vi "read config INI.vi"(8 "error in (no error)":errorcluster, 11 "Cluster in":refnum<vi>) -> (0 "error out":errorcluster, 3 "config.ini value":T1)   [LabVIEW 2014]
uses:
  <vilib>/Utility/config.llb/Read Key (Double).vi
  <vilib>/Utility/config.llb/NI_LVConfig.lvlib
panel:
  # "temperature"
  # "heater"
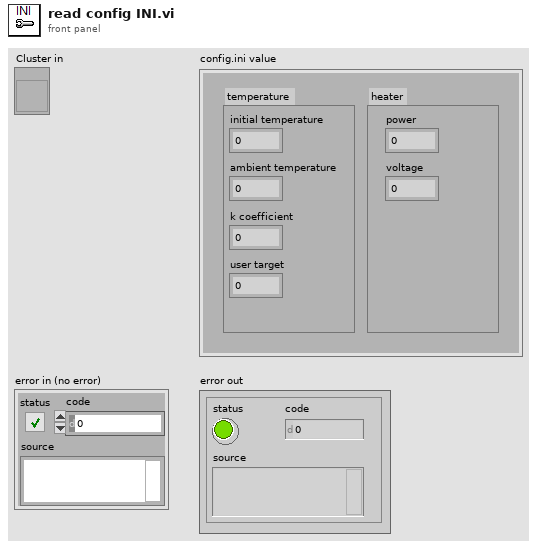
[diagram p1: front panel]
types:
  T1 = cluster{"initial temperature":sgl, "k coefficient":sgl, "ambient temperature":sgl, "user target ":sgl, "power":sgl, "voltage":sgl}
  T2 = typedef "NI_LVConfig.lvlib/Config Data RefNum.ctl" = refnum<k1>
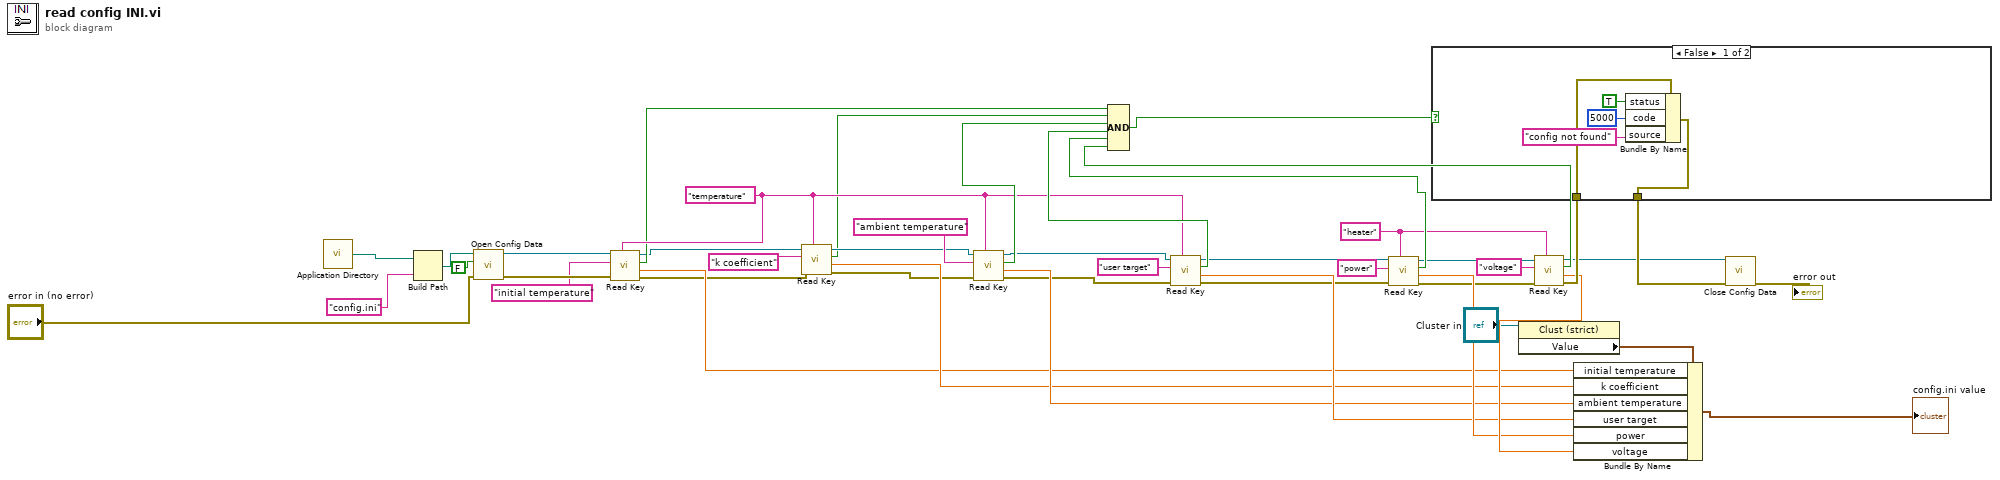
[diagram p0: block diagram]
diagram:
  w25 = "heater" ("section")
  w20 = "temperature" ("section")
  n1 = call <vilib>:"Application Directory.vi"() -> ("Application Directory"=w3:path)
  n2 = Build Path(base path=w3, name or relative path="config.ini") -> (appended path=w4:path)
  n3 = call <vilib>:"Open Config Data.vi"("error in (no error)"="error in (no error)", "create file if necessary (T)"=FALSE, "configuration file path"=w4) -> ("error out"=w10:errorcluster, "refnum"=w5:T2)  [unwired: 6 in, 1 out]
  n4 = call-poly <vilib>:"Read Key.vi"("section"=w20, "error in (no error)"=w10, "key"="initial temperature", "refnum"=w5) -> ("error out"=w11:errorcluster, "value"=w32:dbl, "found?"=w13:bool, "refnum out"=w7:T2)  [unwired: 4 in]
  n5 = call-poly <vilib>:"Read Key.vi"("section"=w20, "error in (no error)"=w11, "key"="k coefficient", "refnum"=w7) -> ("error out"=w17:errorcluster, "value"=w33:dbl, "found?"=w14:bool, "refnum out"=w15:T2)  [unwired: 4 in]
  n6 = call-poly <vilib>:"Read Key.vi"("section"=w20, "error in (no error)"=w17, "key"="ambient temperature", "refnum"=w15) -> ("error out"=w19:errorcluster, "value"=w34:dbl, "found?"=w38:bool, "refnum out"=w18:T2)  [unwired: 4 in]
  n7 = call-poly <vilib>:"Read Key.vi"("section"=w20, "error in (no error)"=w19, "key"="user target", "refnum"=w18) -> ("error out"=w23:errorcluster, "value"=w35:dbl, "found?"=w39:bool, "refnum out"=w22:T2)  [unwired: 4 in]
  n8 = call-poly <vilib>:"Read Key.vi"("section"=w25, "error in (no error)"=w23, "key"="power", "refnum"=w22) -> ("error out"=w28:errorcluster, "value"=w36:dbl, "found?"=w40:bool, "refnum out"=w26:T2)  [unwired: 4 in]
  n9 = property class="Clust (strict)"(reference="Cluster in") -> ("Value"=w30:T1)  [unwired: 1 in, 2 out]
  n10 = call-poly <vilib>:"Read Key.vi"("section"=w25, "error in (no error)"=w28, "key"="voltage", "refnum"=w26) -> ("error out"=w43:errorcluster, "value"=w37:dbl, "found?"=w41:bool, "refnum out"=w29:T2)  [unwired: 4 in]
  n11 = Compound Arithmetic op=AND(w13, w14, w38, w39, w40, w41) -> (w42:bool)
  n12 = case shown="False" w42 {
    tunnel: w43 -> [w50 w51]
    tunnel: [w46 w51] -> w44
    frame False {
      n13 = Bundle By Name(cluster=w50, "status"=TRUE, "code"=5000, "source"="config not found") -> (w46:errorcluster)
    }
    frame True {
    }
  }
  n14 = Bundle By Name(cluster=w30, "initial temperature"=w32, "k coefficient"=w33, "ambient temperature"=w34, "user target"=w35, "power"=w36, "voltage"=w37) -> (→"config.ini value":T1)
  n15 = call <vilib>:"Close Config Data.vi"("error in (no error)"=w44, "refnum"=w29) -> ("error out"=→"error out":errorcluster)  [unwired: 8 in, 1 out]
